vi "PixyCam_Refnum_Registry_Set.vi"(4 "error in (no error)":errorcluster, 6 "refnum name":string, 7 "PixyCamDevRef":T1) -> (0 "error out":errorcluster, 3 "PixyCamDevRef Out":T1)   [LabVIEW 2016, in "PixyCam_LabVIEW.lvlib"]
uses:
  PixyCam_LabVIEW.lvlib
  Private/PixyCam_DevRef.ctl
  Private/PixyCam_SPI_DevRef.ctl
  <vilib>/Rock Robotics/WPI/SPI/WPI_SPIDevRef.ctl
  <vilib>/Rock Robotics/SystemInterfaces/spilib/spi_bus.ctl
  Private/PixyCam_CommMode.ctl
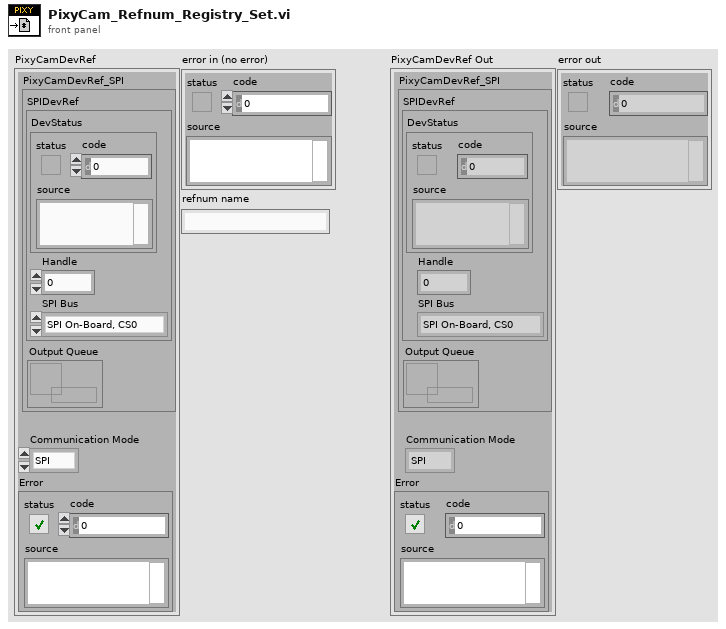
[diagram p1: front panel]
types:
  T1 = typedef "PixyCam_LabVIEW.lvlib/PixyCam_DevRef.ctl" = cluster{"PixyCamDevRef_SPI":T2, "Communication Mode":T5, "Error":errorcluster}
  T2 = typedef "PixyCam_LabVIEW.lvlib/PixyCam_SPI_DevRef.ctl" = cluster{"SPIDevRef":T3, "Output Queue":refnum<queue>}
  T3 = typedef "WPI_SPIDevRef.ctl" = cluster{"DevStatus":errorcluster, "Handle":i32, "SPI Bus":T4}
  T4 = typedef "spi_bus.ctl" = enum16{"SPI On-Board, CS0", "SPI On-Board, CS1", "SPI On-Board, CS2", "SPI On-Board, CS3", "SPI MXP", "Invalid"}
  T5 = typedef "PixyCam_LabVIEW.lvlib/PixyCam_CommMode.ctl" = enum16{"SPI", "I2C", "UART", "Analog", "Digital"}
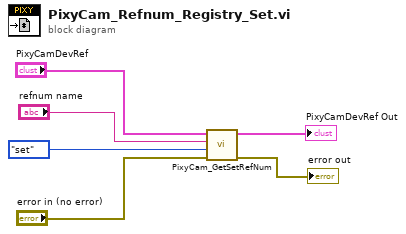
[diagram p0: block diagram]
diagram:
  n1 = call "PixyCam_GetSetRefNum.vi"("error in (no error)"="error in (no error)", "menu"=enum16{"set", "get"}."set", "refnum name"="refnum name", "PixyCamDevRef Set"="PixyCamDevRef") -> ("error out"=→"error out":errorcluster, "PixyCamDevRef Get"=→"PixyCamDevRef Out":T1)  [unwired: 2 in]
